vi "ServerConfigureProcess.vi"(0 "error out":errorcluster caption="error in (no error)", 2 "Process Header":string, 6 "Process Reference in":refnum<vi>, 7 "ConfigFile Reference in":T1 caption="ConfigOut Reference in") -> (3 "entrée d'erreur (pas d'erreur)":errorcluster caption="error out", 9 "ConfigFile Reference out":T1, 10 "Process Reference out":refnum<vi>)   [LabVIEW 2009]
uses:
  <vilib>/Utility/config.llb/Config Data RefNum.ctl
  <vilib>/Utility/config.llb/NI_LVConfig.lvlib
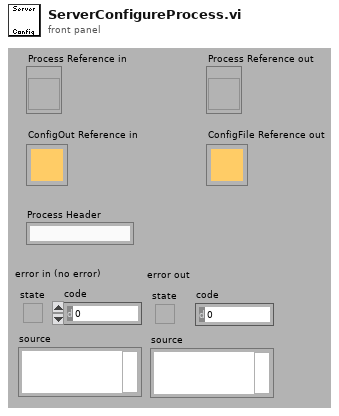
[diagram p1: front panel]
types:
  T1 = typedef "NI_LVConfig.lvlib/Config Data RefNum.ctl" = refnum<k1>
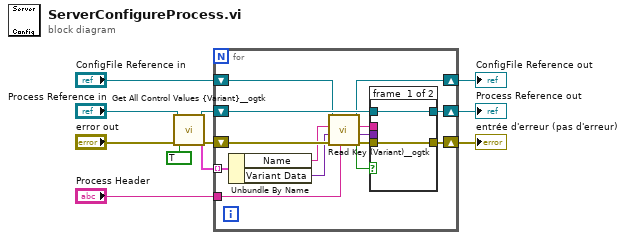
[diagram p0: block diagram]
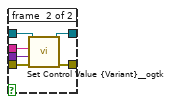
[diagram p2: hidden frame]
diagram:
  n1 = call <userlib>:"Get All Control Values {Variant}__ogtk.vi"("error in (no error)"="error out", "controls (FALSE: indicators)"=TRUE ("controls"), "VI Refnum"="Process Reference in") -> ("error out"=w6:errorcluster, "All Control Values"=w8:cluster{"Name":string, "Variant Data":variant}[], "VI Refnum dup"=w7:refnum<vi>)  [unwired: 6 out]
  n2 = for {
    tunnel: w8 -> [w23] mode=indexing
    shift-right: [w21] -> w10
    shift-left: w6 -> [w24]
    shift-right: [w15] -> w1
    shift-left: "ConfigFile Reference in" -> [w16]
    shift-right: [w14] -> w2
    shift-left: w7 -> [w19]
    tunnel: "Process Header" -> [w13]
    n3 = Unbundle By Name(w23) -> ("Name"=w17:string, "Variant Data"=w22:variant)
    n4 = call <userlib>:"Read Key (Variant)__ogtk.vi"("section"=w13, "error in (no error)"=w24, "type"=w22, "key (optional)"=w17, "refnum"=w16) -> ("error out"=w20:errorcluster, "key-value"=w18:variant, "found?"=w12:bool, "refnum out"=w15:T1)  [unwired: 3 out]
    n5 = case shown="True" w12 {
      tunnel: [w25 w32] -> w21
      tunnel: w20 -> [w25 w31]
      tunnel: w19 -> [w26 w30]
      tunnel: w18 -> [_ w29]
      tunnel: w17 -> [_ w28]
      tunnel: [w26 w27] -> w14
      frame #0 {
      }
      frame #1 {
        n6 = call <userlib>:"Set Control Value {Variant}__ogtk.vi"("error in (no error)"=w31, "Control Name (\"\": use variant name)"=w28, "Value"=w29, "VI Refnum"=w30) -> ("error out"=w32:errorcluster, "VI Refnum dup"=w27:refnum<vi>)  [unwired: 6 out]
      }
    }
  }
  "Process Reference out" <- w2
  "entrée d'erreur (pas d'erreur)" <- w10
  "ConfigFile Reference out" <- w1
